vi "U32 array to U8 array.vi"(11 "Array in":u32[](array[numeric])) -> (3 "Array out":u8[](array[numeric]))   [LabVIEW 2020, in "wamplv.lvlib" / "Utils.lvclass"]
uses:
  Utils.lvclass
  Utils.lvclass/Utils.ctl
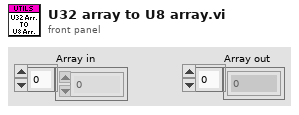
[diagram p1: front panel]
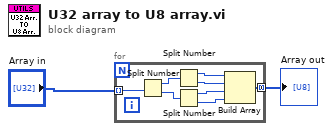
[diagram p0: block diagram]
diagram:
  n1 = for {
    tunnel: "Array in" -> [w10] mode=indexing
    tunnel: [w3] -> w1 mode=concatenating
    n2 = Split Number(x=w10) -> (hi(x)=w9:u16, lo(x)=w8:u16)
    n3 = Split Number(x=w9) -> (hi(x)=w7:u8, lo(x)=w6:u8)
    n4 = Split Number(x=w8) -> (hi(x)=w5:u8, lo(x)=w4:u8)
    n5 = Build Array(w7, w6, w5, w4) -> (w3:u8[])
  }
  "Array out" <- w1
